vi "GetMazeImage.vi"(8 "error in (no error)":errorcluster, 11 "Maze in":refnum<class "Maze.lvclass">) -> (0 "error out":errorcluster, 2 "image data":T1, 3 "Maze out":refnum<class "Maze.lvclass">)   [LabVIEW 2016, in "Maze.lvclass"]
uses:
  Maze.lvclass
  <vilib>/picture/picture.llb/imagedata.ctl
  Maze.lvclass/Maze.ctl
  Room/Room.lvclass
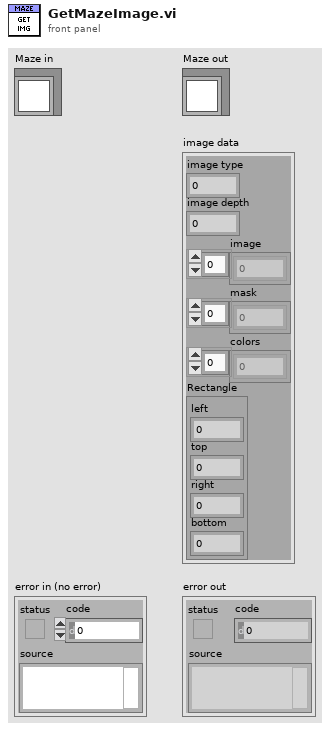
[diagram p1: front panel]
types:
  T1 = typedef "imagedata.ctl" = cluster{"image type":i32, "image depth":i32, "image":u8[], "mask":u8[], "colors":u32[], "Rectangle":cluster{"left":i16, "top":i16, "right":i16, "bottom":i16}}
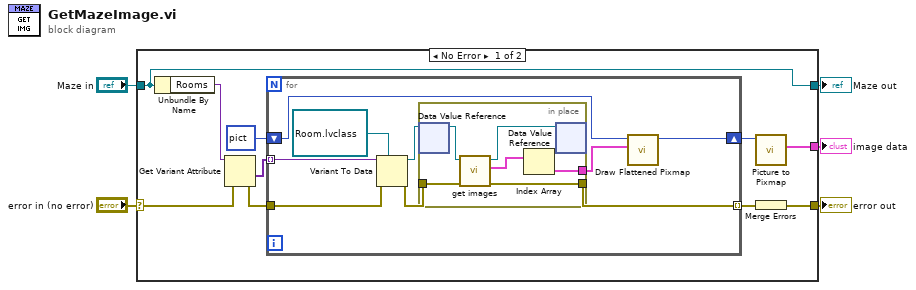
[diagram p0: block diagram]
diagram:
  n1 = case shown="No Error" "error in (no error)" {
    selector: "error in (no error)" -> [w11 w32]
    tunnel: [w8 w32] -> w4
    tunnel: [w15 w31] -> w2
    tunnel: "Maze in" -> [w15 w31]
    tunnel: [w6 _] -> w1
    frame No Error {
      n2 = Unbundle By Name(w15) -> ("Rooms"=w14:variant)
      n3 = Get Variant Attribute(Variant=w14, error in=w11) -> (values=w13:variant[], error out=w12:errorcluster)  [unwired: 2 in, 2 out]
      n4 = for {
        tunnel: w13 -> [w24] mode=indexing
        tunnel: w12 -> [w22]
        shift-right: [w19] -> w7
        shift-left: picture data[5B] ("picture") -> [w20]
        tunnel: [w17] -> w9 mode=indexing
        n5 = Variant To Data(error in=w22, type=refnum<data-value> refnum ("Room*"), Variant=w24) -> (data=w21:refnum<data-value>, error out=w18:errorcluster)
        n6 = in-place {
          in-place-border: [w28] -> w16
          in-place-border: w18 -> [w26]
          in-place-border: [w25] -> w17
          n7 = in-place-dvr #1(w21) -> (w30:refnum<class "Room.lvclass">)  [unwired: 1 out]
          n8 = call-dynamic "get images.vi"("error in (no error)"=w26, "Room in"=w30) -> ("error out"=w25:errorcluster, "images"=w29:T1[], "Room out"=w27:refnum<class "Room.lvclass">)  [unwired: 7 in]
          n9 = Index Array(array=w29) -> (element=w28:T1)  [unwired: 1 in]
          n10 = in-place-dvr #1(w27) -> ()  [unwired: 2 out]
        }
        n11 = call <vilib>:"Draw Flattened Pixmap.vi"("image data"=w16, "picture"=w20) -> ("new picture"=w19:picture)  [unwired: 7 in]
      }
      n12 = call <vilib>:"Picture to Pixmap.vi"("picture"=w7) -> ("image data"=w6:T1)  [unwired: 9 in, 1 out]
      n13 = Merge Errors(w9) -> (w8:errorcluster)
    }
    frame Error {
    }
  }
  "error out" <- w4
  "Maze out" <- w2
  "image data" <- w1
